vi "StateHapticEngine.vi"(0 "Master State In":T1(ring)) -> ()   [LabVIEW 2020]
doc: "Manages the haptic feedback on the driver and manipulator joysticks."
uses:
  GlobalDriverStationData.vi
  GRNF_Joystick.vi
  GlobalAutonomous.vi
  GlobalDriverStationCommands.vi
  GlobalDrivebase.vi
panel:
  in  "Develop New Haptic":bool
  in  "Duty Cycle (%)":dbl=100.0
  in  "Amplitude":dbl=1.0
  in  "Period (s)":dbl=10.0
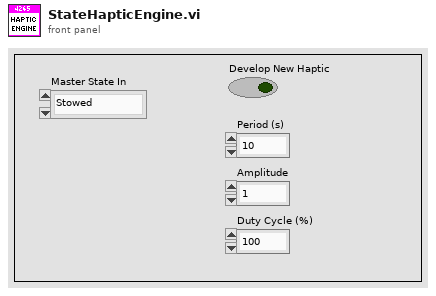
[diagram p1: front panel]
types:
  T1 = enum16{"Stowed", "Balancing", "Scoring", "Hoppering", "Ground", "Shelf"}
  T2 = enum16{"None", "Development", "Longpress Buttons", "End Effector"}
  T3 = typedef "WPI_JoystickDevRef.ctl" = cluster{"Device":T4}
  T4 = typedef "WPI_JoystickDeviceEnum.ctl" = enum16{"USB 0", "USB 1", "USB 2", "USB 3", "USB 4", "USB 5"}
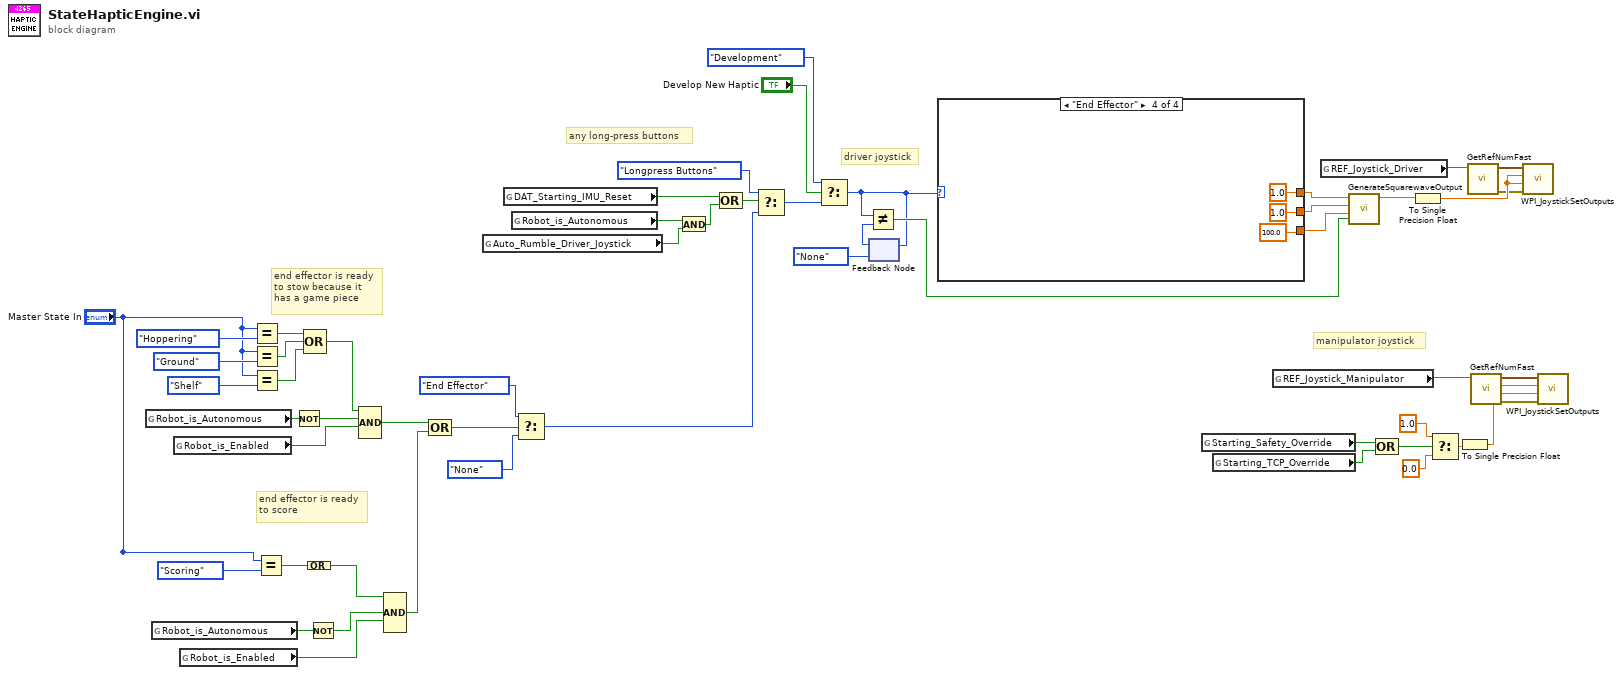
[diagram p0: block diagram]
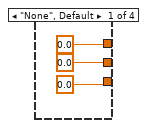
[diagram p2: hidden frame]
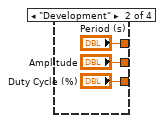
[diagram p3: hidden frame]
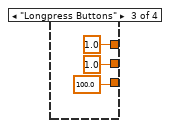
[diagram p4: hidden frame]
diagram:
  # "end effector is ready\nto score"
  # "end effector is ready\nto stow because it\nhas a game piece"
  # "any long-press buttons"
  # "manipulator joystick"
  # "driver joystick"
  n1 = global read "GlobalDriverStationData.vi" "Robot_is_Autonomous"() -> (w28:bool)
  n2 = global read "GlobalDriverStationData.vi" "Robot_is_Autonomous"() -> (w12:bool)
  n3 = global read "GlobalDriverStationData.vi" "Robot_is_Enabled"() -> (w25:bool)
  n4 = global read "GlobalDriverStationData.vi" "Robot_is_Enabled"() -> (w10:bool)
  n5 = Equal?(x="Master State In", y=T1."Hoppering") -> (x = y?=w23:bool)
  n6 = Equal?(x="Master State In", y=T1."Ground") -> (x = y?=w20:bool)
  n7 = Equal?(x="Master State In", y=T1."Shelf") -> (x = y?=w19:bool)
  n8 = Equal?(x="Master State In", y=T1."Scoring") -> (x = y?=w8:bool)
  n9 = Not(x=w28) -> (.not. x?=w27:bool)
  n10 = Compound Arithmetic op=OR(w23, w20, w19) -> (w18:bool)
  n11 = Compound Arithmetic op=OR(w8) -> (w7:bool)
  n12 = Not(x=w12) -> (.not. x?=w11:bool)
  n13 = Compound Arithmetic op=AND(w18, w27, w25) -> (w13:bool, w3:bool)
  n14 = Compound Arithmetic op=AND(w7, w11, w10) -> (w6:bool, w4:bool, w2:bool)
  n15 = Compound Arithmetic op=OR(w13, w6) -> (w5:bool)
  n16 = global read "GlobalAutonomous.vi" "Auto_Rumble_Driver_Joystick"() -> (w46:bool)
  n17 = global read "GlobalDrivebase.vi" "DAT_Starting_IMU_Reset"() -> (w29:bool)
  n18 = global read "GlobalDriverStationData.vi" "Robot_is_Autonomous"() -> (w34:bool)
  n19 = Select(t=T2."End Effector", s=w5, f=T2."None") -> (s? t:f=w26:T2)
  n20 = And(x=w34, y=w46) -> (x .and. y?=w45:bool)
  n21 = Compound Arithmetic op=OR(w29, w45) -> (w43:bool)
  n22 = Select(t=T2."Longpress Buttons", s=w43, f=w26) -> (s? t:f=w32:T2)
  n23 = Select(t=T2."Development", s="Develop New Haptic", f=w32) -> (s? t:f=w38:T2)
  n24 = feedback-in #1(w38) -> ()
  n25 = feedback #1(T2."None") -> (w41:T2)
  n26 = Not Equal?(x=w38, y=w41) -> (x != y?=w40:bool)
  n27 = case shown="\"End Effector\"" w38 {
    tunnel: [0.0 ("Period (s)") "Period (s)" 1.0 ("Period (s)") 1.0 ("Period (s)")] -> w37
    tunnel: [0.0 ("Amplitude") "Amplitude" 1.0 ("Amplitude") 1.0 ("Amplitude")] -> w36
    tunnel: [0.0 ("Duty Cycle (%)") "Duty Cycle (%)" 100.0 ("Duty Cycle (%)") 100.0 ("Duty Cycle (%)")] -> w35
    frame "None", Default {
    }
    frame "Development" {
    }
    frame "Longpress Buttons" {
    }
    frame "End Effector" {
    }
  }
  n28 = global read "GlobalDriverStationData.vi" "Starting_Safety_Override"() -> (w47:bool)
  n29 = global read "GlobalDriverStationData.vi" "Starting_TCP_Override"() -> (w33:bool)
  n30 = global read "GlobalDriverStationCommands.vi" "REF_Joystick_Manipulator"() -> (w31:string)
  n31 = global read "GlobalDriverStationCommands.vi" "REF_Joystick_Driver"() -> (w30:string)
  n32 = call "GenerateSquarewaveOutput.vi"("Init"=w40, "Duty Cycle (%)"=w35, "Amplitude"=w36, "Period (s)"=w37) -> ("Square Wave Ouput"=w44:dbl)  [unwired: 7 in]
  n33 = Compound Arithmetic op=OR(w47, w33) -> (w52:bool)
  n34 = To Single Precision Float(number=w44) -> (single precision float=w57:sgl)
  n35 = Select(t=1.0, s=w52, f=0.0) -> (s? t:f=w54:dbl)
  n36 = To Single Precision Float(number=w54) -> (single precision float=w53:sgl)
  n37 = call-poly "GetRefNumFast.vi"("RefNum Name"=w30) -> ("Error"=w50:errorcluster, "Device Reference"=w51:T3)  [unwired: 5 in]
  n38 = call-poly "GetRefNumFast.vi"("RefNum Name"=w31) -> ("Error"=w49:errorcluster, "Device Reference"=w48:T3)  [unwired: 5 in]
  n39 = call <vilib>:"WPI_JoystickSetOutputs.vi"("error in (no error)"=w50, "Right Rumble"=w57, "Left Rumble"=w57, "JoystickDevRef"=w51) -> ()  [unwired: 6 in, 2 out]
  n40 = call <vilib>:"WPI_JoystickSetOutputs.vi"("error in (no error)"=w49, "Right Rumble"=w53, "Left Rumble"=w53, "JoystickDevRef"=w48) -> ()  [unwired: 6 in, 2 out]
